vi "readI16.vi"(8 "error in (no error)":errorcluster, 11 "ModbusBuffer in":refnum<class "ModbusBufferBuilder.lvclass">) -> (0 "error out":errorcluster, 2 "Output":i16, 3 "ModbusBuffer out":refnum<class "ModbusBufferBuilder.lvclass">)   [LabVIEW 2016, in "ModbusBufferBuilder.lvclass"]
uses:
  ModbusBufferBuilder.lvclass
  ModbusBufferBuilder.lvclass/ModbusBufferBuilder.ctl
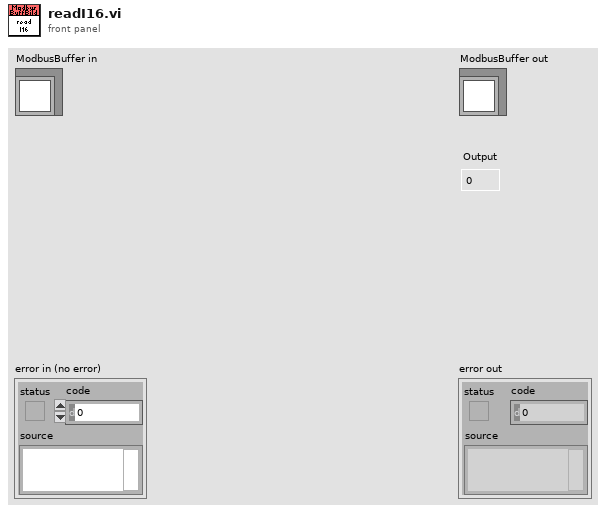
[diagram p1: front panel]
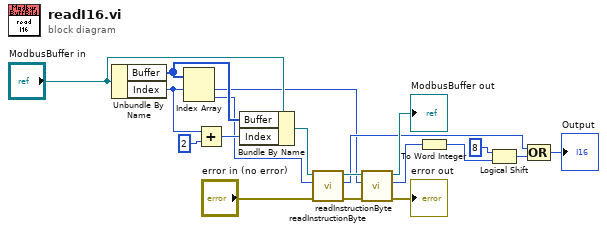
[diagram p0: block diagram]
diagram:
  n1 = Unbundle By Name("ModbusBuffer in") -> ("Buffer"=w18:u16[], "Index"=w15:i32)
  n2 = Index Array(array=w18, index #1=w15) -> (element #1=w2:u16, element #2=w1:u16)  [unwired: 1 in]
  n3 = Add(x=w15, y=2) -> (x+y=w13:i32)
  n4 = Bundle By Name(cluster="ModbusBuffer in", "Buffer"=w18, "Index"=w13) -> (w17:refnum<class "ModbusBufferBuilder.lvclass">)
  n5 = call "readInstructionByte.vi"("error in (no error)"="error in (no error)", "Instruction"=w1, "ModbusBuffer in"=w17) -> ("error out"=w9:errorcluster, "Output"=w10:u8, "ModbusBuffer out"=w12:refnum<class "ModbusBufferBuilder.lvclass">)  [unwired: 6 in]
  n6 = call "readInstructionByte.vi"("error in (no error)"=w9, "Instruction"=w2, "ModbusBuffer in"=w12) -> ("error out"=→"error out":errorcluster, "Output"=w7:u8, "ModbusBuffer out"=→"ModbusBuffer out":refnum<class "ModbusBufferBuilder.lvclass">)  [unwired: 6 in]
  n7 = To Word Integer(number=w7) -> (16bit integer=w6:i16)
  n8 = Logical Shift(y=i16 8, x=w6) -> (x << y=w4:i16)
  n9 = Compound Arithmetic op=OR(w10, w4) -> (→"Output":i16)
